vi "String slicer.vi"(0 "Multiline String":string) -> (1 "Array of numbers with spaces":string[](array[string]), 2 "Array of variable names":string[](array[string]))   [LabVIEW 2013]
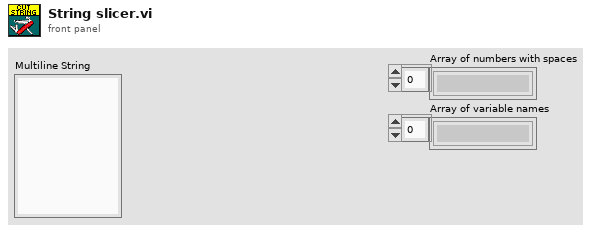
[diagram p1: front panel]
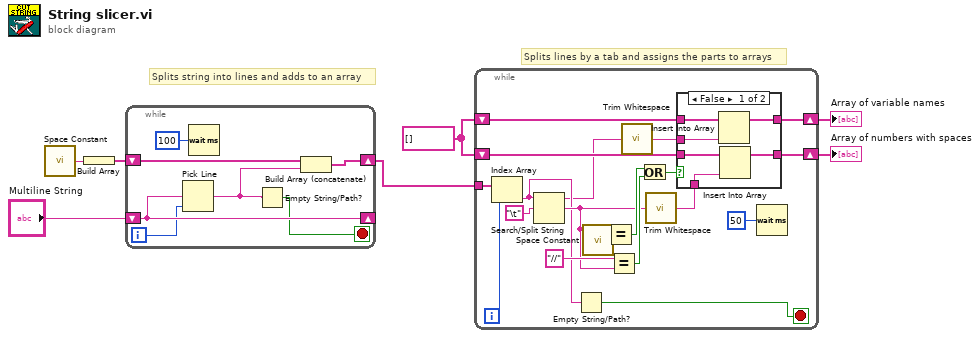
[diagram p0: block diagram]
diagram:
  w2 = string[] []
  # "Splits lines by a tab and assigns the parts to arrays"
  # "Splits string into lines and adds to an array"
  n1 = call <vilib>:"Space Constant.vi"() -> ("String"=w4:string)
  n2 = Build Array(w4) -> (w6:string[])
  n3 = while {
    shift-right: [w14] -> w5
    shift-left: w6 -> [w13]
    shift-right: [w11] -> _
    shift-left: "Multiline String" -> [w11]
    i -> [w10]
    stop <- w8 stop-if-true
    n4 = Pick Line(multi-line string=w11, line index=w10) -> (output string=w9:string)  [unwired: 1 in]
    n5 = Wait (ms)(milliseconds to wait=u32 100) -> ()  [unwired: 1 out]
    n6 = Empty String/Path?(string/path=w9) -> (empty?=w8:bool)
    n7 = Build Array (concatenate)(w13, w9) -> (w14:string[])
  }
  n8 = while {
    shift-right: [w33] -> w3
    shift-left: w2 -> [w32]
    tunnel: w5 -> [w30]
    shift-right: [w21] -> w1
    shift-left: w2 -> [w20]
    i -> [w29]
    stop <- w31 stop-if-true
    n9 = Index Array(array=w30, index=w29) -> (element=w17:string)
    n10 = Search/Split String(string=w17, search string/char (-)="\t") -> (substring before match=w15:string, match + rest of string=w18:string)  [unwired: 1 in, 1 out]
    n11 = Empty String/Path?(string/path=w17) -> (empty?=w31:bool)
    n12 = call <vilib>:"Space Constant.vi"() -> ("String"=w25:string)
    n13 = Equal?(x=w18, y=w25) -> (x = y?=w27:bool)
    n14 = Equal?(x="//", y=w18) -> (x = y?=w26:bool)
    n15 = call <vilib>:"Trim Whitespace.vi"("string"=w15) -> ("trimmed string"=w16:string)  [unwired: 1 in]
    n16 = Or(x=w27, y=w26) -> (x .or. y?=w28:bool)
    n17 = call <vilib>:"Trim Whitespace.vi"("string"=w18) -> ("trimmed string"=w19:string)  [unwired: 1 in]
    n18 = case shown="False" w28 {
      tunnel: [w39 w41] -> w33
      tunnel: w32 -> [w38 w41]
      tunnel: w19 -> [w37 _]
      tunnel: [w36 w40] -> w21
      tunnel: w20 -> [w35 w40]
      tunnel: w16 -> [w34 _]
      frame False {
        n19 = Insert Into Array(array=w35, new element=w34) -> (w36:string[])  [unwired: 1 in]
        n20 = Insert Into Array(array=w38, new element=w37) -> (w39:string[])  [unwired: 1 in]
      }
      frame True {
      }
    }
    n21 = Wait (ms)(milliseconds to wait=u32 50) -> ()  [unwired: 1 out]
  }
  "Array of numbers with spaces" <- w3
  "Array of variable names" <- w1
